vi "About_Time.vi"() -> ()   [LabVIEW 2018]
panel:
  out "error out":errorcluster
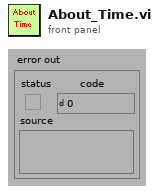
[diagram p1: front panel]
types:
  T1 = enum16{"open", "open or create", "create or replace", "create", "open (read only)"}
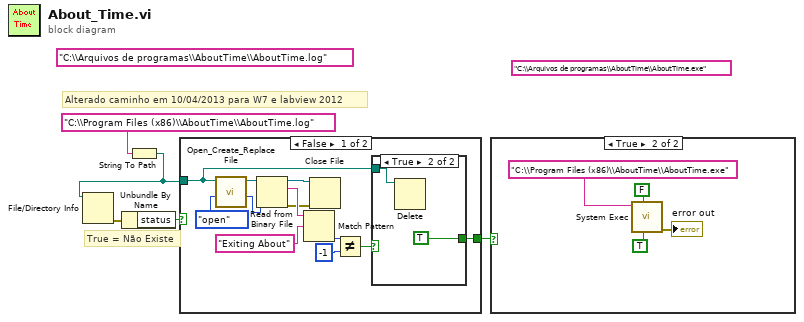
[diagram p0: block diagram]
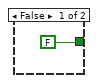
[diagram p3: hidden frame]
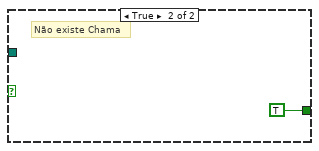
[diagram p4: hidden frame]
diagram:
  (unwired) "C:\\Arquivos de programas\\AboutTime\\AboutTime.exe" ("command line")
  (unwired) "C:\\Arquivos de programas\\AboutTime\\AboutTime.log"
  # "Alterado caminho em 10/04/2013 para W7 e labview 2012"
  # "True = Não Existe"
  n1 = String To Path(string="C:\\Program Files (x86)\\AboutTime\\AboutTime.log") -> (path=w4:path)
  n2 = File/Directory Info(path=w4) -> (error out=w3:errorcluster)  [unwired: 1 in, 6 out]
  n3 = Unbundle By Name(w3) -> ("status"=w2:bool)
  n4 = case shown="False" w2 {
    tunnel: w4 -> [w9 _]
    tunnel: [w8 TRUE] -> w1
    frame False {
      n5 = call <vilib>:"Open_Create_Replace File.vi"("function (open:0)"=T1."open", "file path"=w9) -> ("file size (bytes)"=w15:i32, "refnum"=w16:refnum<file>)  [unwired: 6 in, 2 out]
      n6 = Read from Binary File(10:w15, 11:w16) -> (0:w6:errorcluster, 2:w14:string, 3:w7:refnum<file>)  [unwired: 4 in, 1 out]
      n7 = Match Pattern(string=w14, regular expression="Exiting About") -> (offset past match=w12:i32)  [unwired: 1 in, 3 out]
      n8 = Close File(refnum=w7, error in=w6) -> ()  [unwired: 2 out]
      n9 = Not Equal?(x=w12, y=-1) -> (x != y?=w10:bool)
      n10 = case shown="True" w10 {
        tunnel: w9 -> [_ w20]
        tunnel: [FALSE TRUE] -> w8
        frame False {
        }
        frame True {
          n11 = Delete(path (use dialog)=w20) -> ()  [unwired: 4 in, 3 out]
        }
      }
    }
    frame True {
      # "Não existe Chama"
    }
  }
  n12 = case shown="True" w1 {
    frame False {
    }
    frame True {
      n13 = call <vilib>:"System Exec.vi"("run minimized? (F)"=TRUE, "wait until completion? (T)"=FALSE, "command line"="C:\\Program Files (x86)\\AboutTime\\AboutTime.exe") -> ("error out"=→"error out":errorcluster)  [unwired: 5 in, 3 out]
    }
  }
